vi "Dashboard2.vi"() -> ()   [LabVIEW 2009, in "UI.lvlib"]
uses:
  UI.lvlib
  interface/Pelletron.ctl
  database/Dust Event.ctl
  interface/Dust Info.ctl
  interface/Timetrace.ctl
  interface/Data Source.ctl
  interface/Dust Head.ctl
  interface/Interface.lvlib
  database/Data Store.lvclass
  waveform/Waveform.lvlib
  database/Database.lvlib
panel:
  in  "stop":bool
  out "Dust Source Queue Status":bool
  out "Dust Event Queue Status":bool
  out "Pelletron Queue Status":bool
  in  "Tab Control":T1(tab)=enum."Dust Event Queue"
  out "Pelletron\nQueue Depth":i32
  out "Last Pelletron Data Tick":T2
  out "Pelletron Queue Error":errorcluster
  out "Pelletron\nElements Handled":i32
  in  "Path for HDF5 Files":path=path "C:/data"
  out "Dust Queue Error":errorcluster
  out "Last HDF5 File Written":string
  out "Last Event Posted to Database":T3
  out "Last Dust Trace":T4
  out "Dust Events\nHandled":i32
  out "Dust Event\nQueue Depth":i32
  in  "Use Dust Source Queue?":bool
  in  "Source Settings (manual)":T7
  out "Dust Source Data":T7
  out "Dust Source Error":errorcluster
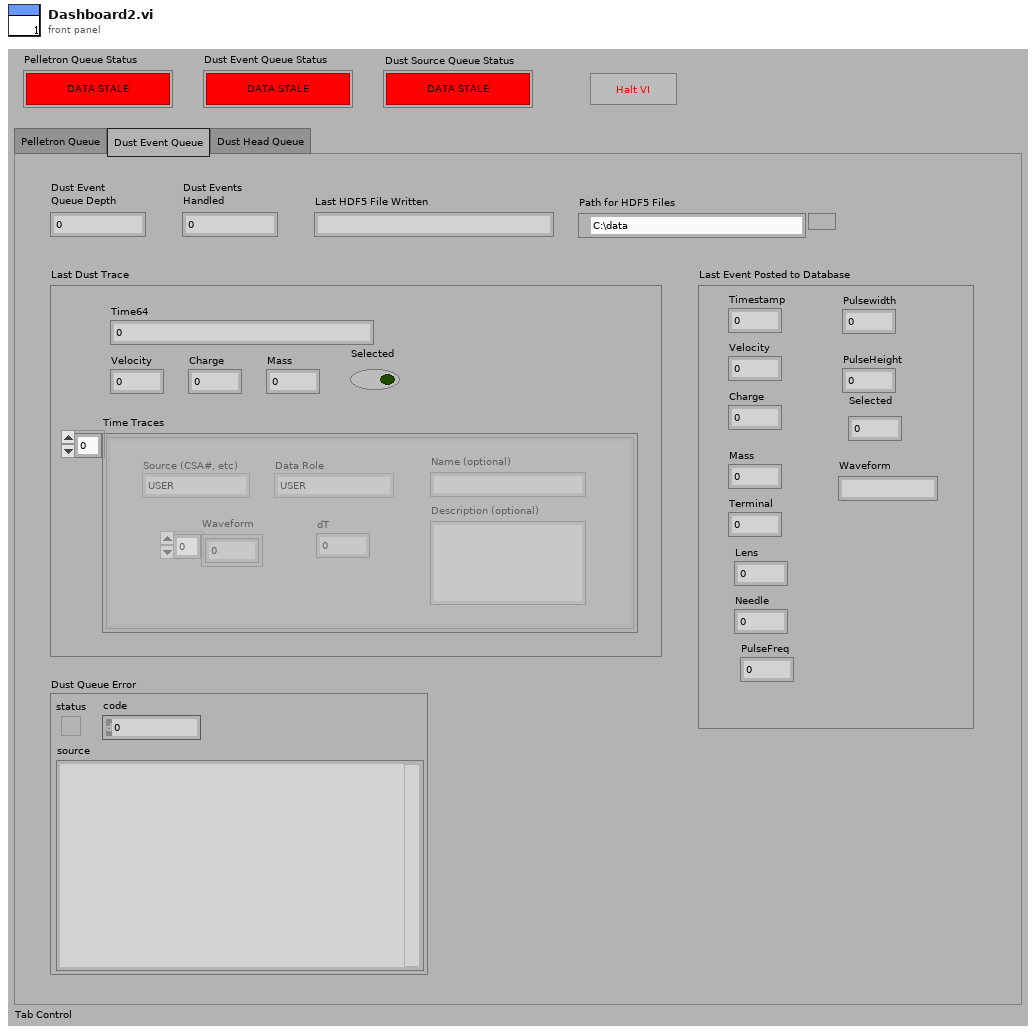
[diagram p1: front panel]
types:
  T1 = enum32{"Pelletron Queue", "Dust Event Queue", "Dust Head Queue"}
  T2 = typedef "Interface.lvlib/Pelletron.ctl" = cluster{"Timestamp":u64, "High Voltage":sgl, "Vacuum Pressure":sgl, "Column Current":sgl, "Chain Current":sgl, "- High Voltage Supply":dbl, "+ High Voltage Supply":dbl, "Radiation":dbl, "Lost Charge":dbl, "Control High Voltage":dbl, "HV Control Difference":dbl}
  T3 = typedef "Database.lvlib/Dust Event.ctl" = cluster{"Timestamp":u64, "Velocity":sgl, "Charge":sgl, "Mass":sgl, "Terminal":sgl, "Lens":sgl, "Needle":sgl, "PulseFreq":sgl, "Pulsewidth":dbl, "PulseHeight":sgl, "Selected":i8, "Waveform":string}
  T4 = typedef "Interface.lvlib/Dust Info.ctl" = cluster{"Time64":u64, "Velocity":dbl, "Charge":dbl, "Mass":dbl, "Time Traces":T5[], "Selected":bool}
  T5 = typedef "Interface.lvlib/Timetrace.ctl" = cluster{"Source (CSA#, etc)":T6, "Data Role":enum16{"USER", "FIRST DETECTOR", "SECOND DETECTOR", "THIRD DETECTOR", "FINAL DETECTOR"}, "Waveform":sgl[], "dT":sgl, "Name (optional)":string, "Description (optional)":string}
  T6 = typedef "Interface.lvlib/Data Source.ctl" = enum16{"USER", "CSA1", "CSA2", "CSA3", "CSA4", "CSA5", "CSA6", ""}
  T7 = typedef "Interface.lvlib/Dust Head.ctl" = cluster{"Lens":dbl, "Needle/Housing":dbl, "Pulse Frequency":dbl, "Pulse Height":dbl, "Pulse Width":dbl}
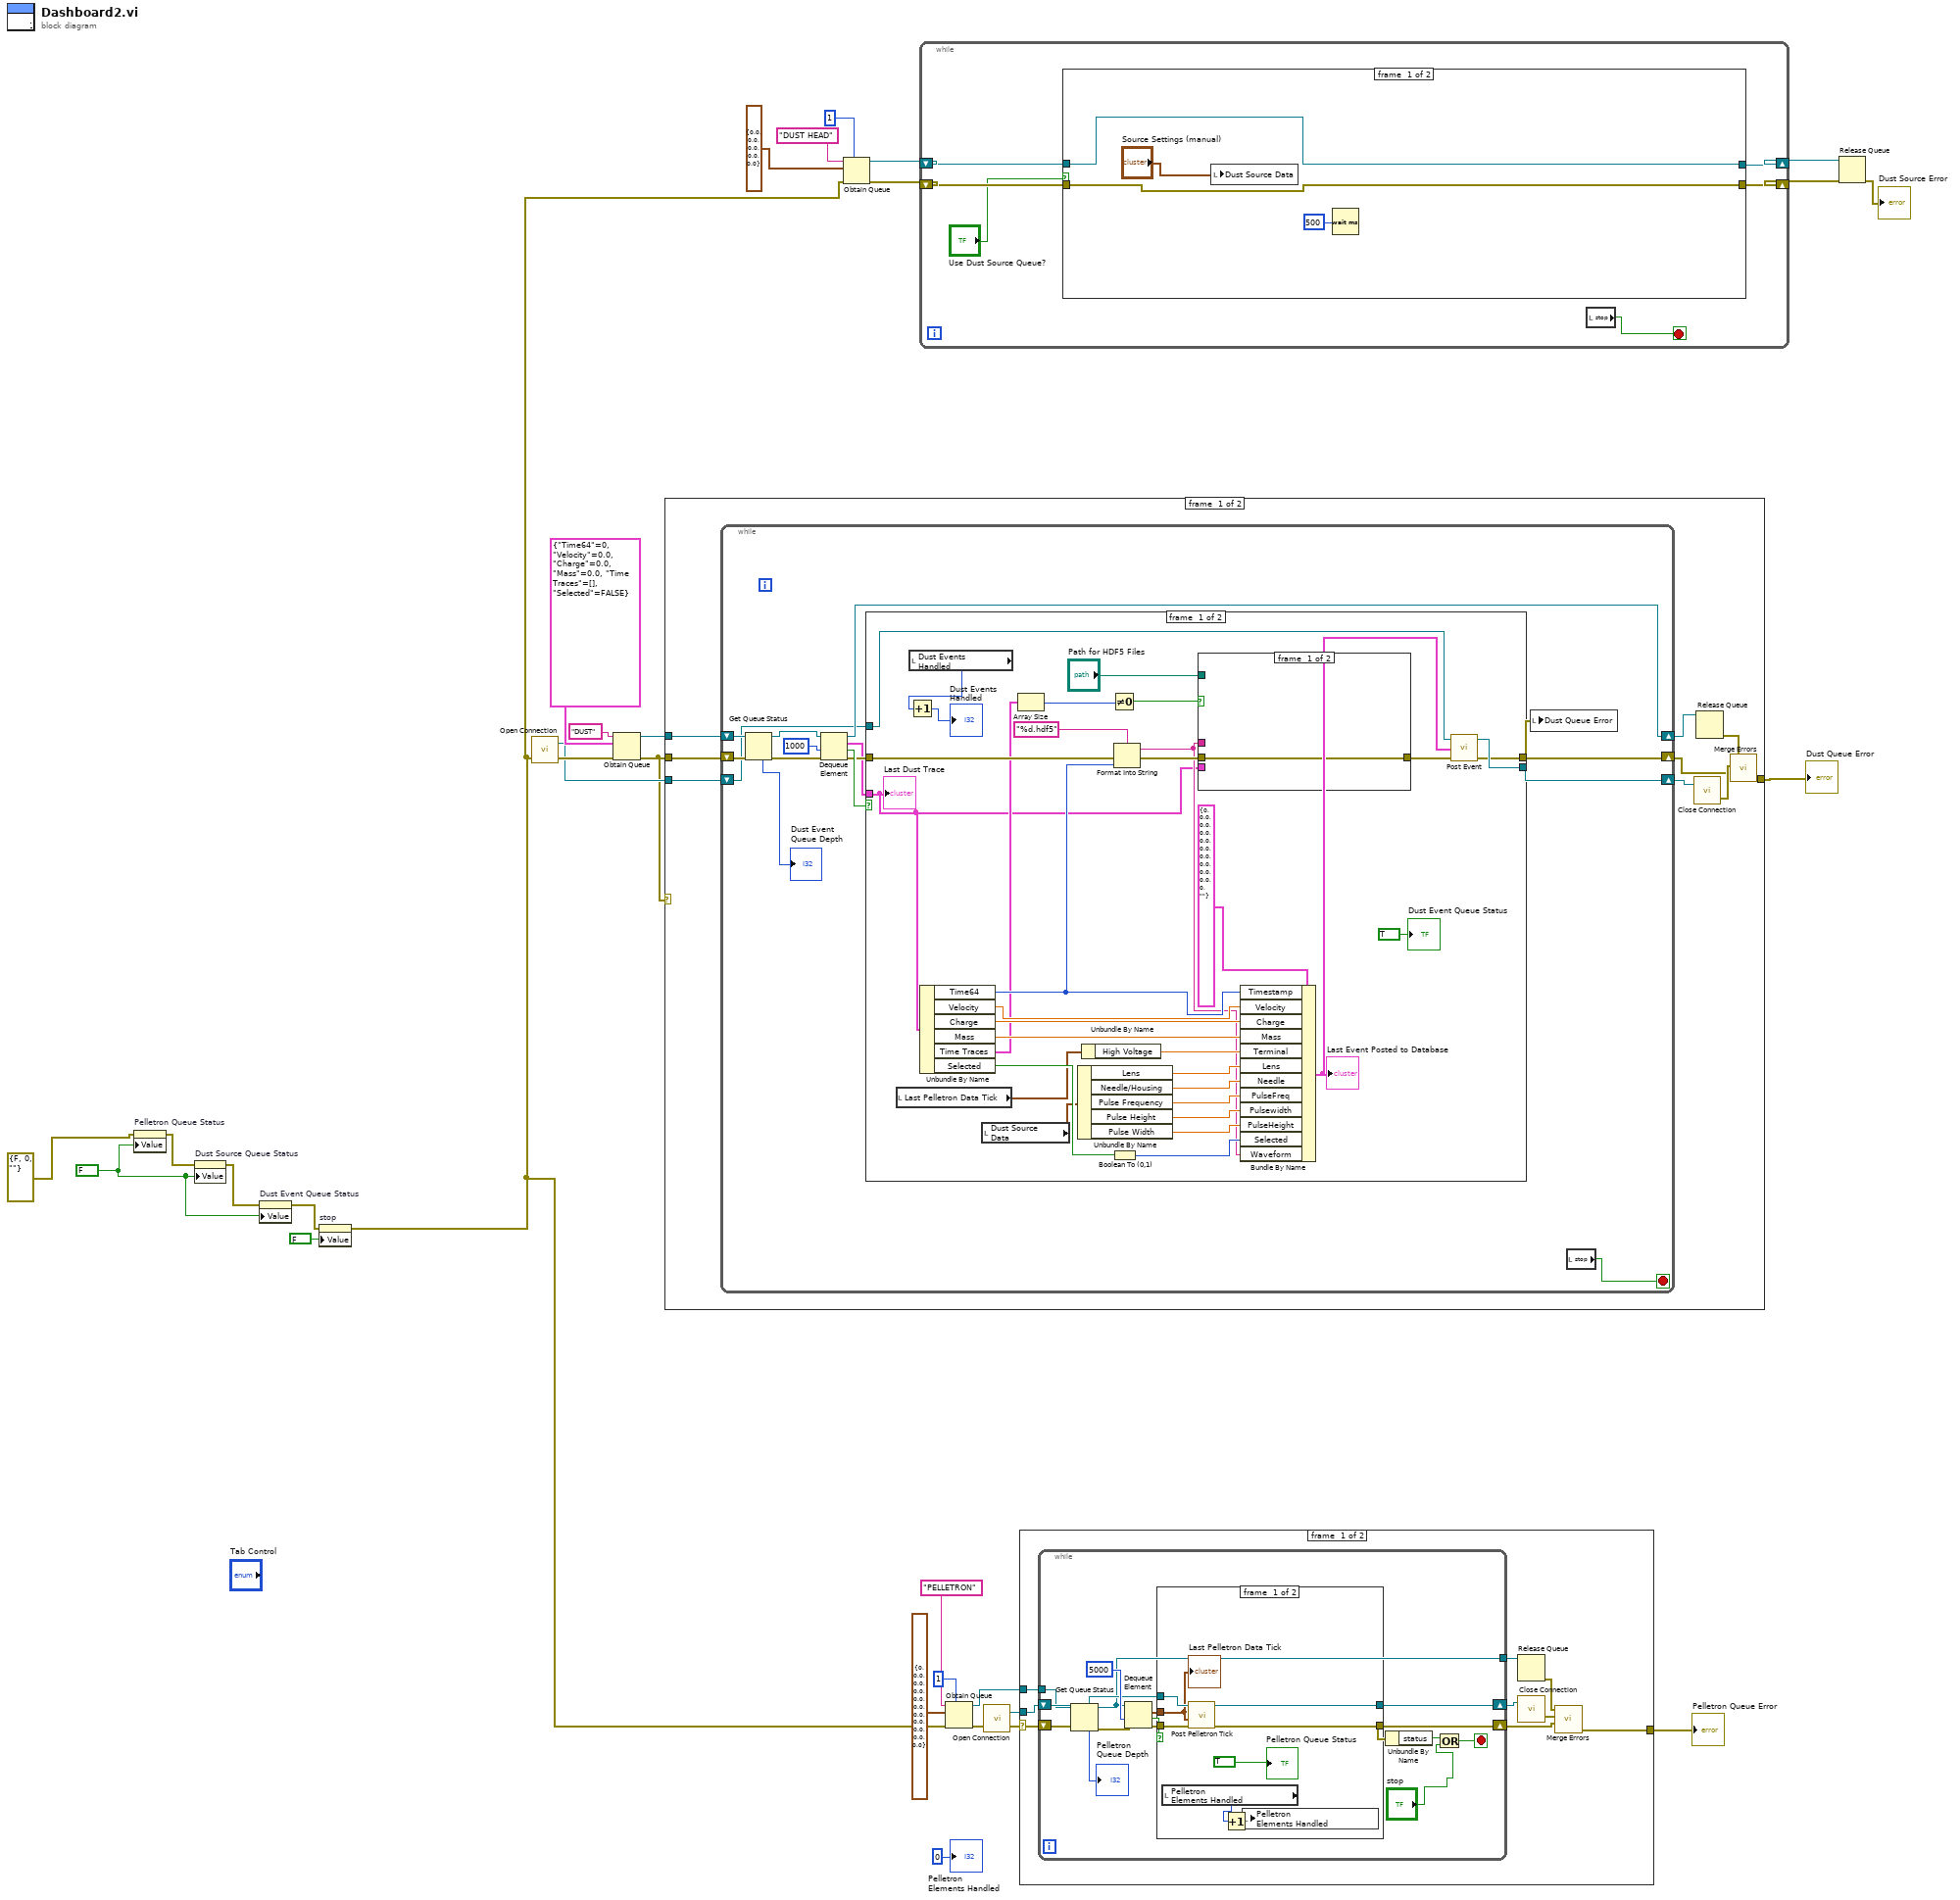
[diagram p0: block diagram]
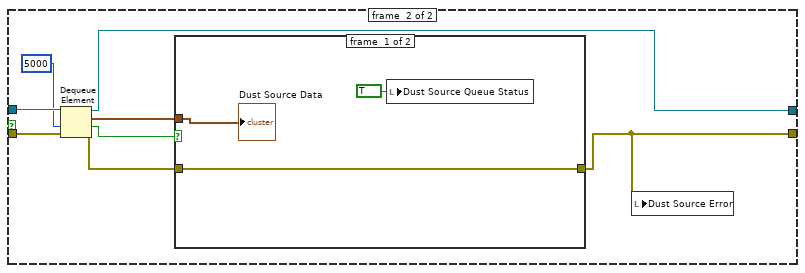
[diagram p2: hidden frame]
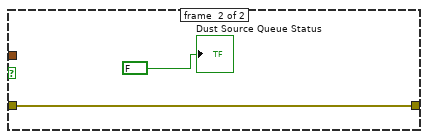
[diagram p3: hidden frame]
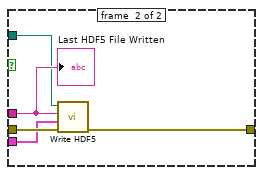
[diagram p4: hidden frame]
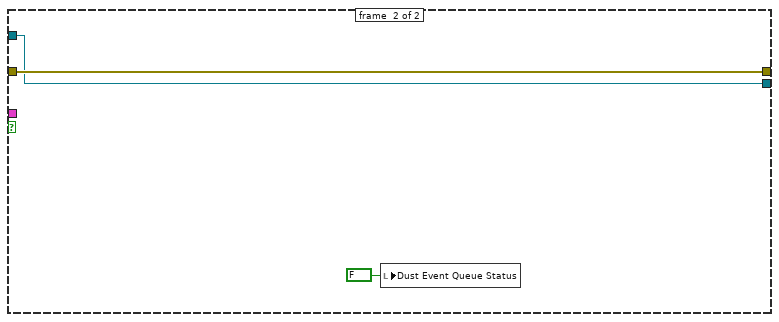
[diagram p5: hidden frame]
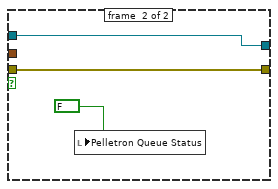
[diagram p7: hidden frame]
diagram:
  w2 = FALSE ("Pelletron Queue Status")
  n1 = property on="Pelletron Queue Status" class="Bool (strict)"(error in=errorcluster {"status"=FALSE, "code"=0, "source"=""} ("error in (no error)"), "Value"=w2) -> (error out=w6:errorcluster)  [unwired: 1 in, 1 out]
  n2 = property on="Dust Source Queue Status" class="Bool (strict)"(error in=w6, "Value"=w2) -> (error out=w5:errorcluster)  [unwired: 1 in, 1 out]
  n3 = property on="Dust Event Queue Status" class="Bool (strict)"(error in=w5, "Value"=w2) -> (error out=w4:errorcluster)  [unwired: 1 in, 1 out]
  n4 = property on="stop" class="Bool (strict)"(error in=w4, "Value"=FALSE ("stop")) -> (error out=w3:errorcluster)  [unwired: 1 in, 1 out]
  n5 = call "Open Connection.vi"("error in (no error)"=w3) -> ("error out"=w20:errorcluster, "Database.lvlib:Data Store.lvclass"=w19:refnum<class "Data Store.lvclass">)  [unwired: 1 in]
  n6 = Obtain Queue(name (unnamed)="DUST", element data type=T4 {"Time64"=0, "Velocity"=0.0, "Charge"=0.0, "Mass"=0.0, "Time Traces"=[], "Selected"=FALSE} ("Cluster"), error in (no error)=w20) -> (queue out=w21:refnum<queue>, error out=w18:errorcluster)  [unwired: 2 in, 1 out]
  n7 = case shown="No Error" w18 {
    tunnel: w21 -> [w40 _]
    tunnel: w18 -> [w39 w96]
    tunnel: w19 -> [w37 _]
    tunnel: [w35 w96] -> w17
    frame #0 {
      n8 = while {
        shift-right: [w46] -> w38
        shift-left: w40 -> [w51]
        shift-right: [w44] -> w32
        shift-left: w39 -> [w49]
        shift-right: [w42] -> w36
        shift-left: w37 -> [w43]
        stop <- w41 stop-if-true
        n9 = Get Queue Status(queue=w51, error in (no error)=w49) -> (queue out=w50:refnum<queue>, error out=w48:errorcluster, # elements in queue=→"Dust Event\nQueue Depth":i32)  [unwired: 1 in, 5 out]
        n10 = Dequeue Element(queue=w50, timeout in ms (-1)=1000, error in (no error)=w48) -> (queue out=w46:refnum<queue>, element=w45:T4, timed out?=w53:bool, error out=w52:errorcluster)
        n11 = case shown="False" w53 {
          tunnel: w52 -> [w72 w95]
          tunnel: [w68 w95] -> w44
          tunnel: w45 -> [w62 _]
          tunnel: w43 -> [w71 w94]
          tunnel: [w69 w94] -> w42
          frame #0 {
            n12 = local read "Last Pelletron Data Tick"() -> (w59:T2)
            n13 = local read "Dust Events\nHandled"() -> (w58:i32)
            n14 = Increment(x=w58) -> (x+1=→"Dust Events\nHandled":i32)
            n15 = Unbundle By Name(w62) -> ("Time64"=w73:u64, "Velocity"=w86:dbl, "Charge"=w85:dbl, "Mass"=w84:dbl, "Time Traces"=w64:T5[], "Selected"=w82:bool)
            n16 = local read "Dust Source Data"() -> (w80:T7)
            n17 = Array Size(array=w64) -> (size(s)=w67:i32)
            n18 = Unbundle By Name(w80) -> ("Lens"=w79:dbl, "Needle/Housing"=w78:dbl, "Pulse Frequency"=w77:dbl, "Pulse Height"=w76:dbl, "Pulse Width"=w75:dbl)
            n19 = Unbundle By Name(w59) -> ("High Voltage"=w83:sgl)
            n20 = Not Equal To 0?(x=w67) -> (x != 0?=w66:bool)
            n21 = Boolean To (0,1)(Boolean=w82) -> (0, 1=w81:i16)
            n22 = Format Into String(format string="%d.hdf5", error in=w72, w73) -> (resulting string=w63:string, error out=w65:errorcluster)  [unwired: 1 in]
            n23 = case shown="True" w66 {
              tunnel: w65 -> [w87 w92]
              tunnel: w62 -> [_ w90]
              tunnel: [w87 w91] -> w61
              tunnel: w63 -> [_ w89]
              tunnel: "Path for HDF5 Files" -> [_ w88]
              frame #0 {
              }
              frame #1 {
                n24 = call "Write HDF5.vi"("error in (no error)"=w92, "Cluster"=w90, "Filename"=w89, "Path"=w88) -> ("error out"=w91:errorcluster)  [unwired: 7 in]
                "Last HDF5 File Written" <- w89
              }
            }
            n25 = Bundle By Name(cluster=T3 {"Timestamp"=0, "Velocity"=0.0, "Charge"=0.0, "Mass"=0.0, "Terminal"=0.0, "Lens"=0.0, "Needle"=0.0, "PulseFreq"=0.0, "Pulsewidth"=0.0, "PulseHeight"=0.0, "Selected"=0, "Waveform"=""} ("Cluster"), "Timestamp"=w73, "Velocity"=w86, "Charge"=w85, "Mass"=w84, "Terminal"=w83, "Lens"=w79, "Needle"=w78, "PulseFreq"=w77, "Pulsewidth"=w76, "PulseHeight"=w75, "Selected"=w81, "Waveform"=w63) -> (w70:T3)
            "Last Event Posted to Database" <- w70
            n26 = call "Post Event.vi"("error in (no error)"=w61, "Event In"=w70, "Database.lvlib:Data Store.lvclass"=w71) -> ("error out"=w68:errorcluster, "Database.lvlib:Data Store.lvclass 2"=w69:refnum<class "Data Store.lvclass">)  [unwired: 1 in]
            "Last Dust Trace" <- w62
            "Dust Event Queue Status" <- TRUE ("Dust Event\nQueue Status")
          }
          frame #1 {
            n27 = local write "Dust Event Queue Status"(FALSE ("Dust Event\nQueue Status")) -> ()
          }
        }
        n28 = local write "Dust Queue Error"(w44) -> ()
        n29 = local read "stop"() -> (w41:bool)
      }
      n30 = call "Close Connection.vi"("Database.lvlib:Data Store.lvclass"=w36) -> ("error out"=w33:errorcluster)  [unwired: 2 in]
      n31 = Release Queue(queue=w38) -> (error out=w34:errorcluster)  [unwired: 2 in, 2 out]
      n32 = call <vilib>:"Merge Errors.vi"("error in 3 (no error)"=w32, "error in 2 (no error)"=w33, "error in 1 (no error)"=w34) -> ("error out"=w35:errorcluster)  [unwired: 4 in]
    }
    frame #1 {
    }
  }
  "Dust Queue Error" <- w17
  n33 = Obtain Queue(max queue size (-1, unlimited)=1, name (unnamed)="DUST HEAD", element data type=T7 {"Lens"=0.0, "Needle/Housing"=0.0, "Pulse Frequency"=0.0, "Pulse Height"=0.0, "Pulse Width"=0.0} ("Cluster"), error in (no error)=w3) -> (queue out=w11:refnum<queue>, error out=w12:errorcluster)  [unwired: 1 in, 1 out]
  n34 = while {
    shift-right: [w100] -> w10
    shift-left: w11 -> [w101]
    shift-right: [w99] -> w9
    shift-left: w12 -> [w102]
    stop <- w98 stop-if-true
    n35 = case shown="True" "Use Dust Source Queue?" {
      tunnel: w102 -> [w103 w114]
      tunnel: w101 -> [w104 w113]
      tunnel: [w104 w108] -> w100
      tunnel: [w103 w107] -> w99
      frame #0 {
        n36 = local write "Dust Source Data"("Source Settings (manual)") -> ()
        n37 = Wait (ms)(milliseconds to wait=u32 500) -> ()  [unwired: 1 out]
      }
      frame #1 {
        n38 = Dequeue Element(queue=w113, timeout in ms (-1)=5000, error in (no error)=w114) -> (queue out=w108:refnum<queue>, element=w109:T7, timed out?=w111:bool, error out=w110:errorcluster)
        n39 = case shown="False" w111 {
          tunnel: w110 -> [w116 w119]
          tunnel: [w116 w119] -> w107
          tunnel: w109 -> [w115 _]
          frame #0 {
            n40 = local write "Dust Source Queue Status"(TRUE ("Dust Head update status")) -> ()
            "Dust Source Data" <- w115
          }
          frame #1 {
            "Dust Source Queue Status" <- FALSE ("Dust Head update status")
          }
        }
        n41 = local write "Dust Source Error"(w107) -> ()
      }
    }
    n42 = local read "stop"() -> (w98:bool)
  }
  n43 = Obtain Queue(max queue size (-1, unlimited)=1, name (unnamed)="PELLETRON", element data type=T2 {"Timestamp"=0, "High Voltage"=0.0, "Vacuum Pressure"=0.0, "Column Current"=0.0, "Chain Current"=0.0, "- High Voltage Supply"=0.0, "+ High Voltage Supply"=0.0, "Radiation"=0.0, "Lost Charge"=0.0, "Control High Voltage"=0.0, "HV Control Difference"=0.0} ("Cluster"), error in (no error)=w3) -> (queue out=w29:refnum<queue>, error out=w30:errorcluster)  [unwired: 1 in, 1 out]
  n44 = call "Open Connection.vi"("error in (no error)"=w30) -> ("error out"=w27:errorcluster, "Database.lvlib:Data Store.lvclass"=w28:refnum<class "Data Store.lvclass">)  [unwired: 1 in]
  n45 = case shown="No Error" w27 {
    selector: w27 -> [w126 w155]
    tunnel: w29 -> [w128 _]
    tunnel: w28 -> [w127 _]
    tunnel: [w120 w155] -> w25
    frame #0 {
      n46 = while {
        tunnel: w128 -> [w133]
        shift-right: [w138] -> w124
        shift-left: w127 -> [w139]
        shift-right: [w136] -> w121
        shift-left: w126 -> [w134]
        tunnel: [w132] -> w125
        stop <- w137 stop-if-true
        n47 = Get Queue Status(queue=w133, error in (no error)=w134) -> (queue out=w132:refnum<queue>, error out=w135:errorcluster, # elements in queue=→"Pelletron\nQueue Depth":i32)  [unwired: 1 in, 5 out]
        n48 = Dequeue Element(queue=w132, timeout in ms (-1)=5000, error in (no error)=w135) -> (element=w140:T2, timed out?=w141:bool, error out=w142:errorcluster)  [unwired: 1 out]
        n49 = case shown="False" w141 {
          tunnel: w142 -> [w151 w154]
          tunnel: w140 -> [w147 _]
          tunnel: w139 -> [w150 w153]
          tunnel: [w149 w154] -> w136
          tunnel: [w148 w153] -> w138
          frame #0 {
            n50 = local read "Pelletron\nElements Handled"() -> (w146:i32)
            n51 = call "Post Pelletron Tick.vi"("error in (no error)"=w151, "Pelletron data"=w147, "Database.lvlib:Data Store.lvclass"=w150) -> ("error out"=w149:errorcluster, "Database.lvlib:Data Store.lvclass 2"=w148:refnum<class "Data Store.lvclass">)  [unwired: 7 in]
            n52 = Increment(x=w146) -> (x+1=w145:i32)
            n53 = local write "Pelletron\nElements Handled"(w145) -> ()
            "Last Pelletron Data Tick" <- w147
            "Pelletron Queue Status" <- TRUE ("Data Status")
          }
          frame #1 {
            n54 = local write "Pelletron Queue Status"(FALSE ("Data Status")) -> ()
          }
        }
        n55 = Unbundle By Name(w136) -> ("status"=w130:bool)
        n56 = Or(x=w130, y="stop") -> (x .or. y?=w137:bool)
      }
      n57 = Release Queue(queue=w125) -> (error out=w123:errorcluster)  [unwired: 2 in, 2 out]
      n58 = call "Close Connection.vi"("Database.lvlib:Data Store.lvclass"=w124) -> ("error out"=w122:errorcluster)  [unwired: 2 in]
      n59 = call <vilib>:"Merge Errors.vi"("error in 3 (no error)"=w121, "error in 2 (no error)"=w122, "error in 1 (no error)"=w123) -> ("error out"=w120:errorcluster)  [unwired: 4 in]
    }
    frame #1 {
    }
  }
  "Pelletron Queue Error" <- w25
  n60 = Release Queue(queue=w10, error in (no error)=w9) -> (error out=→"Dust Source Error":errorcluster)  [unwired: 1 in, 2 out]
  "Pelletron\nElements Handled" <- 0 ("Elements\nHandled")
